vi "ziModGetByteArray.vi"(8 "Error In":errorcluster, 10 "ModResults":T2, 11 "ModHandle In":T5 {"ModHandle" format="0x%08x"; "Conn" format="0x%08x"}) -> (0 "Error Out":errorcluster, 2 "ByteArray":T1[](array[typedef]), 3 "ModHandle Out":T5 {"ModHandle" format="0x%08x"; "Conn" format="0x%08x"})   [LabVIEW 2009, in "Zurich Instruments LabOne.lvlib"]
doc: "Use this vi to get ByteArrayData from a ModResult returned from ziModGetNextNode.vi. \nIt returns an array of BytesArrays."
uses:
  <instrlib>/Zurich Instruments LabOne/Zurich Instruments LabOne.lvlib
  <instrlib>/Zurich Instruments LabOne/Public/Modules/ziTypeModHandle.ctl
  <instrlib>/Zurich Instruments LabOne/Public/Modules/ziTypeModResults.ctl
  <instrlib>/Zurich Instruments LabOne/Public/Data/ziTypePollType.ctl
  <instrlib>/Zurich Instruments LabOne/Public/Modules/ziTypeModGenericHeader.ctl
  <instrlib>/Zurich Instruments LabOne/Public/Data/ziTypeByteArray.ctl
  <instrlib>/Zurich Instruments LabOne/Private/ziLV32.dll
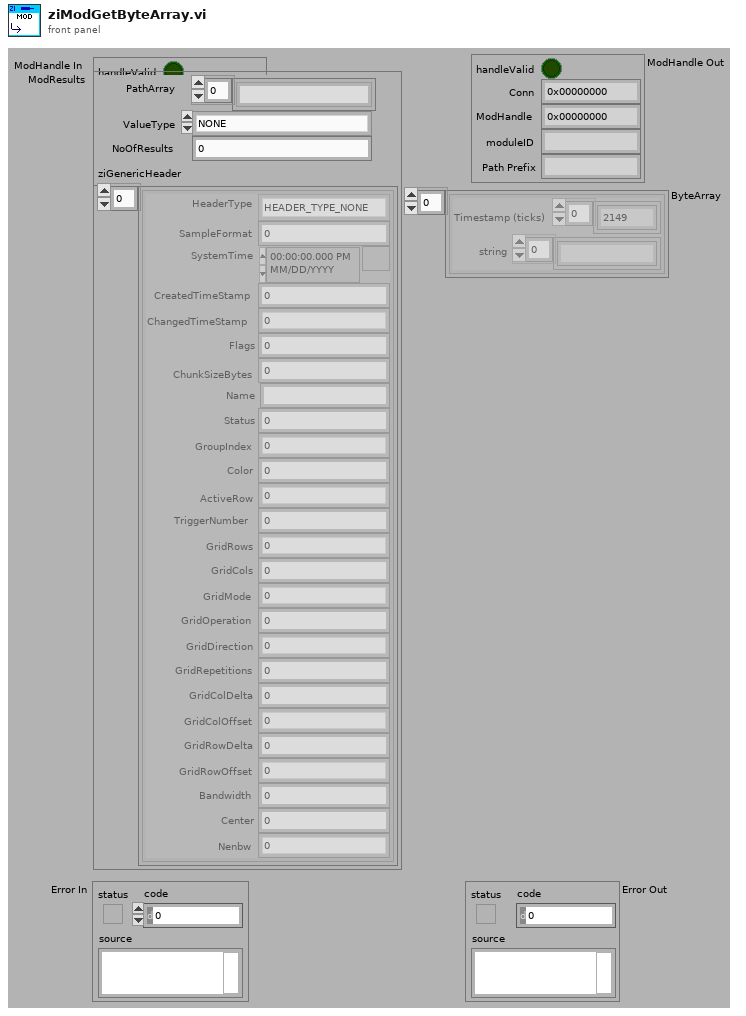
[diagram p1: front panel]
types:
  T1 = typedef "Zurich Instruments LabOne.lvlib/ziTypeByteArray.ctl" = cluster{"Timestamp (ticks)":u64[], "string":string[]}
  T2 = typedef "Zurich Instruments LabOne.lvlib/ziTypeModResults.ctl" = cluster{"PathArray":string[], "ValueType":T3, "NoOfResults":u64, "ziGenericHeader":T4[]}
  T3 = typedef "Zurich Instruments LabOne.lvlib/ziTypePollType.ctl" = enum16{"NONE", "DOUBLE_DATA", "INTEGER_DATA", "DEMOD_SAMPLE", "SCOPE_WAVE_HF2", "AUXIN_SAMPLE", "DIO_SAMPLE", "BYTE_ARRAY", "PWA_WAVE", "9", "10", "11", "12", "13", "14", "15", "TREE_CHANGE_DEPRI", "17", "ERROR", "19", "20", "21", "22", "23", "24", "25", "26", "27", "28", "29", "30", "31", "DOUBLE_DATA_TS", "INTEGER_DATA_TS", "34", "SCOPE_WAVE", "SCOPE_WAVE_EX", "37", "BYTE_ARRAY_TS", "39", "40", "41", "42", "43", "44", "45", "CNT_DATA", "47", "TREE_CHANGE", "49", "50", "51", "52", "53", "54", "55", "56", "57", "58", "59", "60", "61", "62", "63", "SWEEPER_DATA", "SPECTRUM_DATA", "ADVISOR_DATA", "VECTOR_DATA", "IMP_DATA"}
  T4 = typedef "Zurich Instruments LabOne.lvlib/ziTypeModGenericHeader.ctl" = cluster{"HeaderType":enum8{"HEADER_TYPE_NONE", "HEADER_TYPE_SWTRIGGER", "HEADER_TYPE_SWEEPER"}, "SampleFormat":u8, "SystemTime":timestamp, "CreatedTimeStamp":u64, "ChangedTimeStamp":u64, "Flags":u32, "ChunkSizeBytes":u64, "Name":string, "Status":u32, "GroupIndex":u32, "Color":u32, "ActiveRow":u32, "TriggerNumber":u64, "GridRows":u32, "GridCols":u32, "GridMode":u32, "GridOperation":u32, "GridDirection":u32, "GridRepetitions":u32, "GridColDelta":dbl, "GridColOffset":dbl, "GridRowDelta":dbl, "GridRowOffset":dbl, "Bandwidth":dbl, "Center":dbl, "Nenbw":dbl}
  T5 = typedef "Zurich Instruments LabOne.lvlib/ziTypeModHandle.ctl" = cluster{"handleValid":bool, "Conn":u64, "ModHandle":u64, "moduleID":string, "Path Prefix":string}
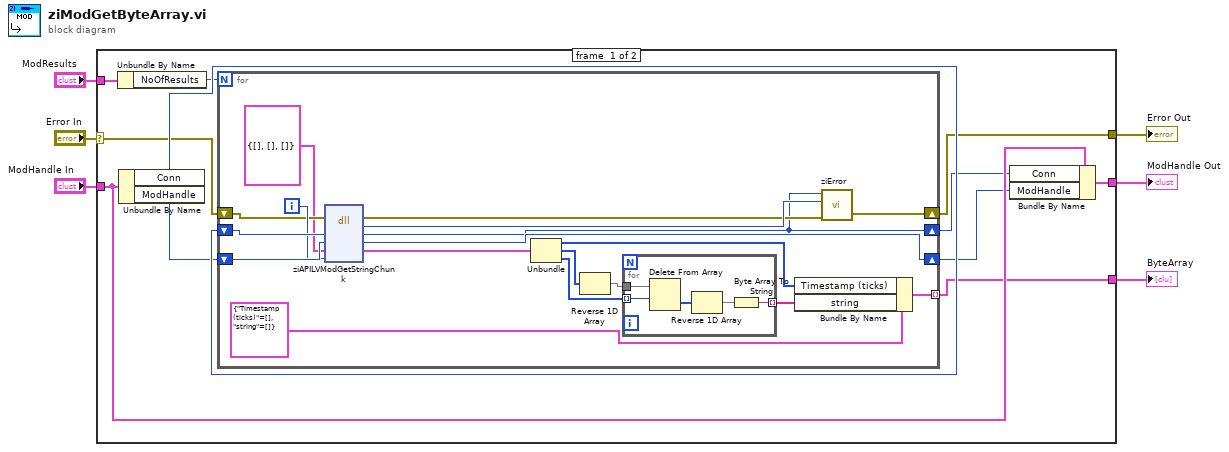
[diagram p0: block diagram]
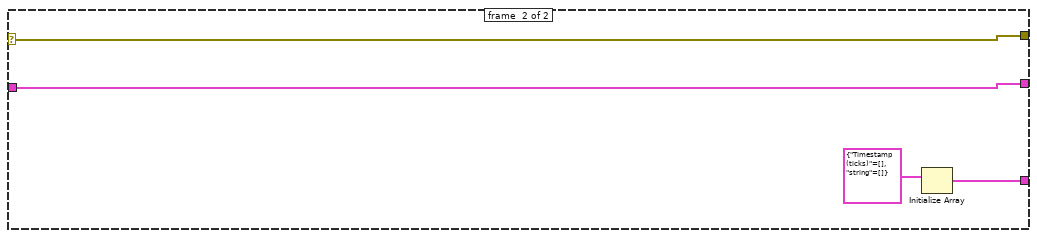
[diagram p2: hidden frame]
diagram:
  n1 = case shown="No Error" "Error In" {
    selector: "Error In" -> [w8 w43]
    tunnel: [w9 w43] -> w2
    tunnel: [w16 w44] -> w5
    tunnel: "ModHandle In" -> [w17 w44]
    tunnel: "ModResults" -> [w13 _]
    tunnel: [w7 w42] -> w1
    frame #0 {
      n2 = Unbundle By Name(w13) -> ("NoOfResults"=w12:u64)
      n3 = Unbundle By Name(w17) -> ("Conn"=w15:u64, "ModHandle"=w14:u64)
      n4 = for {
        N: w12 -> [_]
        tunnel: [w19] -> w7 mode=indexing
        shift-right: [w31] -> w9
        shift-left: w8 -> [w28]
        shift-right: [w27] -> w11
        shift-left: w15 -> [w34]
        shift-right: [w35] -> w10
        shift-left: w14 -> [w33]
        i -> [w32]
        n5 = dll-call lib="C:/Program Files (x86)/National Instruments/LabVIEW 2009/instr.lib/Zurich Instruments LabOne/Private/ziLV*.*" fn="ziAPILVModGetStringChunk" label="ziAPILVModGetSweeperWaveChunk"(error in=w28, "Conn"=w34, "ModHandle"=w33, "ByteArray"=cluster{u64[], u8[], u64[]} {[], [], []}, "chunk_idx"=w32) -> (error out=w29:errorcluster, "return type"=w30:u32, "Conn"=w27:u64, "ModHandle"=w35:u64, "ByteArray"=w20:cluster{u64[], u8[], u64[]})  [unwired: 3 in, 1 out]
        n6 = Unbundle(w20) -> (w21:u64[], w22:u8[], w25:u64[])
        n7 = Reverse 1D Array(array=w22) -> (reversed array=w24:u8[])
        n8 = for {
          tunnel: w25 -> [w38] mode=indexing
          tunnel: w24 -> [w39]
          tunnel: [w40] -> w23 mode=indexing
          n9 = Delete From Array(array=w39, length=w38) -> (deleted portion=w37:u8[])  [unwired: 1 in, 1 out]
          n10 = Reverse 1D Array(array=w37) -> (reversed array=w36:u8[])
          n11 = Byte Array To String(unsigned byte array=w36) -> (string=w40:string)
        }
        n12 = Bundle By Name(cluster=T1 {"Timestamp (ticks)"=[], "string"=[]} ("ByteArray"), "Timestamp (ticks)"=w21, "string"=w23) -> (w19:T1)
        n13 = call <instrlib>:"ziError.vi"("Conn"=w27, "ziErrorCode"=w30, "Error In"=w29) -> ("Error Out"=w31:errorcluster)  [unwired: 2 in, 1 out]
      }
      n14 = Bundle By Name(cluster=w17, "Conn"=w11, "ModHandle"=w10) -> (w16:T5)
    }
    frame #1 {
      n15 = Initialize Array(T1 {"Timestamp (ticks)"=[], "string"=[]} ("ByteArray")) -> (w42:T1[])  [unwired: 1 in]
    }
  }
  "Error Out" <- w2
  "ModHandle Out" <- w5
  "ByteArray" <- w1
